vi "flush_avg_queues.vi"(2 "Combo Box":string(combo), 7 "avg_Q_data in":T1) -> (8 "avg_Q_data out":T1)   [LabVIEW 2023]
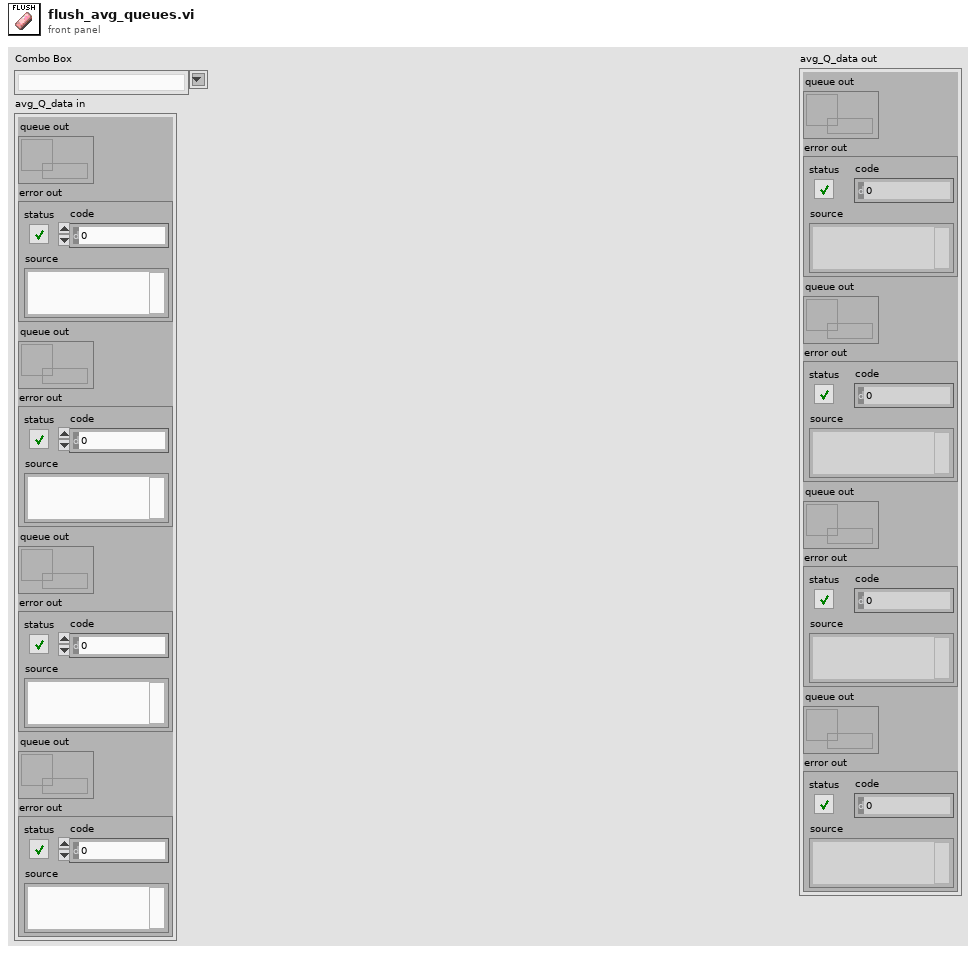
[diagram p1: front panel]
types:
  T1 = cluster{"queue out":refnum<queue>, "error out":errorcluster, "queue out":refnum<queue>, "error out":errorcluster, "queue out":refnum<queue>, "error out":errorcluster, "queue out":refnum<queue>, "error out":errorcluster}
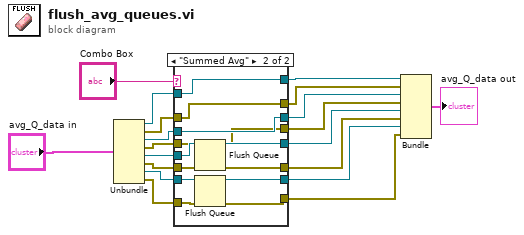
[diagram p0: block diagram]
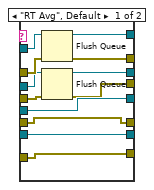
[diagram p2: hidden frame]
diagram:
  n1 = Unbundle("avg_Q_data in") -> ("queue out"=w18:refnum<queue>, "error out"=w17:errorcluster, "queue out"=w16:refnum<queue>, "error out"=w15:errorcluster, "queue out"=w14:refnum<queue>, "error out"=w13:errorcluster, "queue out"=w12:refnum<queue>, "error out"=w11:errorcluster)
  n2 = case shown="\"Summed Avg\"" "Combo Box" {
    tunnel: w18 -> [w31 w35]
    tunnel: w17 -> [w30 w34]
    tunnel: w16 -> [w29 w33]
    tunnel: w15 -> [w28 w32]
    tunnel: w14 -> [w27 w43]
    tunnel: w13 -> [w26 w42]
    tunnel: w12 -> [w25 w41]
    tunnel: w11 -> [w24 w40]
    tunnel: [w27 w39] -> w5
    tunnel: [w26 w38] -> w4
    tunnel: [w25 w37] -> w3
    tunnel: [w24 w36] -> w2
    tunnel: [w23 w35] -> w9
    tunnel: [w22 w34] -> w8
    tunnel: [w21 w33] -> w7
    tunnel: [w20 w32] -> w6
    frame "RT Avg", Default {
      n3 = Flush Queue(queue=w31, error in (no error)=w30) -> (queue out=w23:refnum<queue>, error out=w22:errorcluster)  [unwired: 1 out]
      n4 = Flush Queue(queue=w29, error in (no error)=w28) -> (queue out=w21:refnum<queue>, error out=w20:errorcluster)  [unwired: 1 out]
    }
    frame "Summed Avg" {
      n5 = Flush Queue(queue=w43, error in (no error)=w42) -> (queue out=w39:refnum<queue>, error out=w38:errorcluster)  [unwired: 1 out]
      n6 = Flush Queue(queue=w41, error in (no error)=w40) -> (queue out=w37:refnum<queue>, error out=w36:errorcluster)  [unwired: 1 out]
    }
  }
  n7 = Bundle("queue out"=w9, "error out"=w8, "queue out"=w7, "error out"=w6, "queue out"=w5, "error out"=w4, "queue out"=w3, "error out"=w2) -> (→"avg_Q_data out":T1)  [unwired: 1 in]
